vi "jsonParseFloat.vi"(8 "error in (no error)":errorcluster, 9 "default":sgl, 10 "path":string, 11 "d in":i64) -> (0 "error out":errorcluster, 1 "found?":bool, 2 "value":sgl, 3 "d out":i64)   [LabVIEW 2015, in "rapidjson wrapper.lvlib"]
uses:
  rapidjson wrapper.lvlib
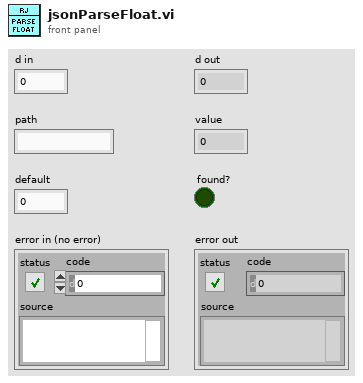
[diagram p1: front panel]
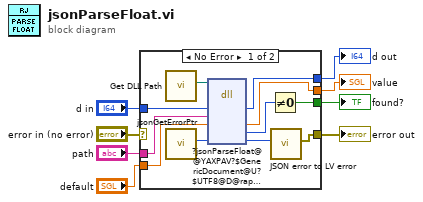
[diagram p0: block diagram]
diagram:
  n1 = case shown="No Error" "error in (no error)" {
    selector: "error in (no error)" -> [_ w22]
    tunnel: [w17 w22] -> w8
    tunnel: [w14 w21] -> w6
    tunnel: "default" -> [w15 w21]
    tunnel: [w13 w20] -> w4
    tunnel: "d in" -> [w12 w20]
    tunnel: "path" -> [w11 _]
    tunnel: [w9 _] -> w1
    frame No Error {
      n2 = call "Get DLL Path.vi"() -> ("Path"=w19:path)  [unwired: 11 in]
      n3 = call "jsonGetErrorPtr.vi"() -> ("return type"=w16:i64)  [unwired: 10 in, 1 out]
      n4 = dll-call lib="C:/Users/tblair/Documents/Git Projects/rapidjson-for-LabVIEW/lvrjs/Debug/lvrjs.dll" fn="?jsonParseFloat@@YAXPAV?$GenericDocument@U?$UTF8@D@rapidjson@@V?$MemoryPoolAllocator@VCrtAllocator@rapidjson@@@2@VCrtAllocator@2@@rapidjson@@PADAAMAA_N0@Z"(path in=w19, "d"=w12, "path"=w11, "value"=w15, "jsonError"=w16) -> ("d"=w13:i64, "value"=w14:sgl, "result"=w10:i32, "jsonError"=w18:i64)  [unwired: 5 in, 2 out]
      n5 = Not Equal To 0?(x=w10) -> (x != 0?=w9:bool)
      n6 = call "JSON error to LV error.vi"("jsonError"=w18) -> ("error out"=w17:errorcluster)  [unwired: 10 in]
    }
    frame Error {
    }
  }
  "error out" <- w8
  "value" <- w6
  "d out" <- w4
  "found?" <- w1
